vi "Dev List - Remove DTRow.vi"(7 "Row Index":i32, 8 "error in (no error)":errorcluster, 9 "Dev Data Lookup Table in":variant, 10 "DataGridView in":refnum<class "DataGridView.lvclass">, 11 "Controller UI in":refnum<class "Controller UI.lvclass">) -> (0 "error out":errorcluster, 1 "Dev Data Lookup Table in out":variant, 2 "DataGridView out":refnum<class "DataGridView.lvclass">)   [LabVIEW 2016, in "Controller UI.lvlib" / "Controller UI.lvclass"]
uses:
  <userlib>/Common Components/Controller UI/Controller UI.lvclass
  C:/Program Files (x86)/National Instruments/LabVIEW 2016/vi.lib/ActorFramework/Actor/Actor.lvclass
  <userlib>/LabVIEWdotNetDataGrid/source/DataGridView/DataGridView.lvclass
  <userlib>/Common Components/Hardware/DevInfo/DevInfo.lvclass
  <vilib>/ActorFramework/Actor/Actor.lvclass/Actor.ctl
  <userlib>/Common Components/Hardware/DevInfo/DevInfo.lvclass/DevInfo.ctl
  <userlib>/Common Components/Controller/Messages/Remove a Dev Requested by UI Msg/Remove a Dev Requested by UI Msg.lvclass/Remove a Dev Requested by UI Msg.ctl
  <vilib>/ActorFramework/Message Enqueuer/Message Enqueuer.lvclass/Message Enqueuer.ctl
  <userlib>/Common Components/Hardware/DevInfo/Read GUID.vi
  <vilib>/ActorFramework/Message Enqueuer/Enqueue.vi
  <userlib>/Common Components/Controller/Messages/Remove a Dev Requested by UI Msg/Remove a Dev Requested by UI Msg.lvclass
  C:/Program Files (x86)/National Instruments/LabVIEW 2016/vi.lib/ActorFramework/Message/Message.lvclass
  <userlib>/LabVIEWdotNetDataGrid/source/DataGridView/Get DataRow (String).vi
  <vilib>/ActorFramework/Message Priority Queue/Priority Enqueue.vi
  <vilib>/ActorFramework/Actor/Actor.lvclass
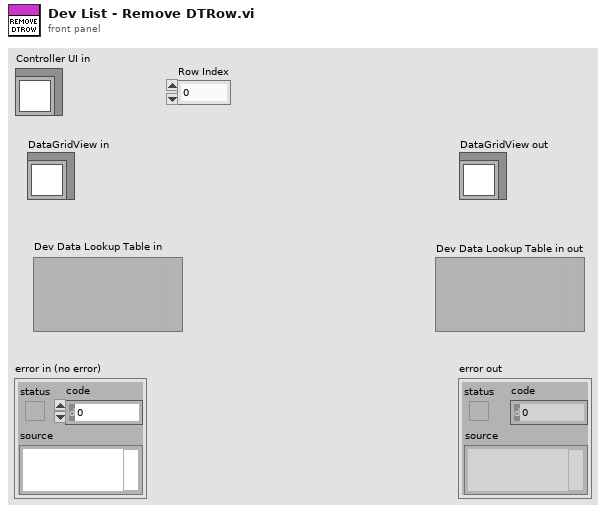
[diagram p1: front panel]
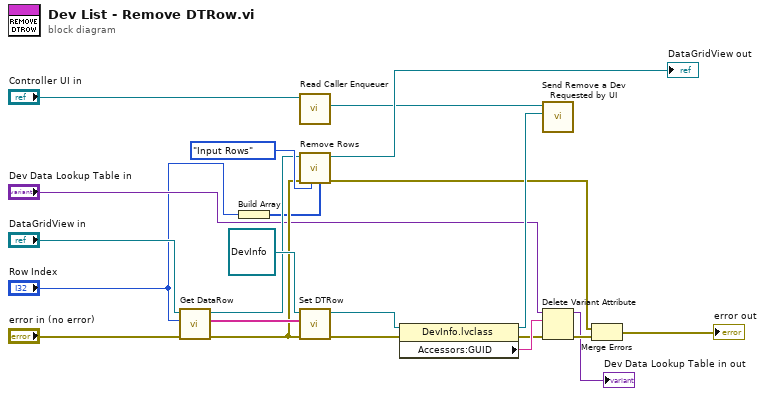
[diagram p0: block diagram]
diagram:
  n1 = call-poly <userlib>:"Get DataRow.vi"("error in (no error)"="error in (no error)", "index"="Row Index", "DataGridView in"="DataGridView in") -> ("error out"=w15:errorcluster, "Array"=w19:string[], "DataGridView out"=w20:refnum<class "DataGridView.lvclass">)  [unwired: 6 in]
  n2 = Build Array("Row Index") -> (w1:i32[])
  n3 = call <vilib>:"Read Caller Enqueuer.vi"("Actor"="Controller UI in") -> ("Caller Enqueuer"=w3:refnum<class "Message Enqueuer.lvclass">)  [unwired: 10 in]
  n4 = call <userlib>:"Remove Rows.vi"("Rows"=w1, "Mode"=enum16{"Selected Rows", "Input Rows"}."Input Rows", "error in (no error)"=w15, "DataGridView in"=w20) -> ("error out"=w14:errorcluster, "DataGridView out"=→"DataGridView out":refnum<class "DataGridView.lvclass">)  [unwired: 6 in]
  n5 = call <userlib>:"Set DTRow.vi"("error in (no error)"=w15, "Dev Row Elements"=w19, "DevInfo in"=refnum<class "DevInfo.lvclass"> refnum ("DevInfo")) -> ("error out"=w13:errorcluster, "DevInfo out"=w18:refnum<class "DevInfo.lvclass">)  [unwired: 7 in]
  n6 = property class="DevInfo.lvclass"(reference=w18, error in=w13) -> (reference out=w17:refnum<class "DevInfo.lvclass">, error out=w12:errorcluster, "Accessors:GUID"=w16:string)
  n7 = call <userlib>:"Send Remove a Dev Requested by UI.vi"("DevInfo"=w17, "Message Enqueuer in"=w3) -> ()  [unwired: 8 in, 2 out]
  n8 = Delete Variant Attribute(4:w12, 6:w16, 7:"Dev Data Lookup Table in") -> (0:w11:errorcluster, 3:→"Dev Data Lookup Table in out":variant)  [unwired: 1 out]
  n9 = Merge Errors(w14, w11) -> (→"error out":errorcluster)
